vi "GSP_Manager_GT_driver.vi"(4 "error in (no error)":errorcluster, 5 "Grating # (Move Only)":i32, 6 "Action":T1) -> (0 "error out":errorcluster, 3 "reference out (launch only)":refnum<vi>)   [LabVIEW 2015]
doc: "Provides an interface to the Grating Translation Manager. See the actions below.\n\nLaunch - launch the manager thread supplying references to the controls that the thread will update.\n\nHome - Home the grating translation stage\n\nMove - Move the grating to the position supplied by Grating#\n\nShutdown - Shutdown the grating translation manager"
uses:
  GTdriveractions.ctl
  SystemUtil/Command.ctl
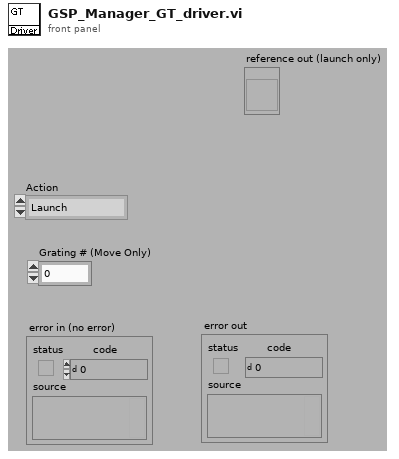
[diagram p1: front panel]
types:
  T1 = typedef "GTdriveractions.ctl" = enum16{"Launch", "INIT_CTL", "Move", "Home", "Shutdown"}
  T2 = typedef "Command.ctl" = cluster{"Command":string, "Parameter":string}
  T3 = cluster{string, "type string":i16[], "data string":string}
  T4 = cluster{string, "type string":i16[], "data string":string}[]
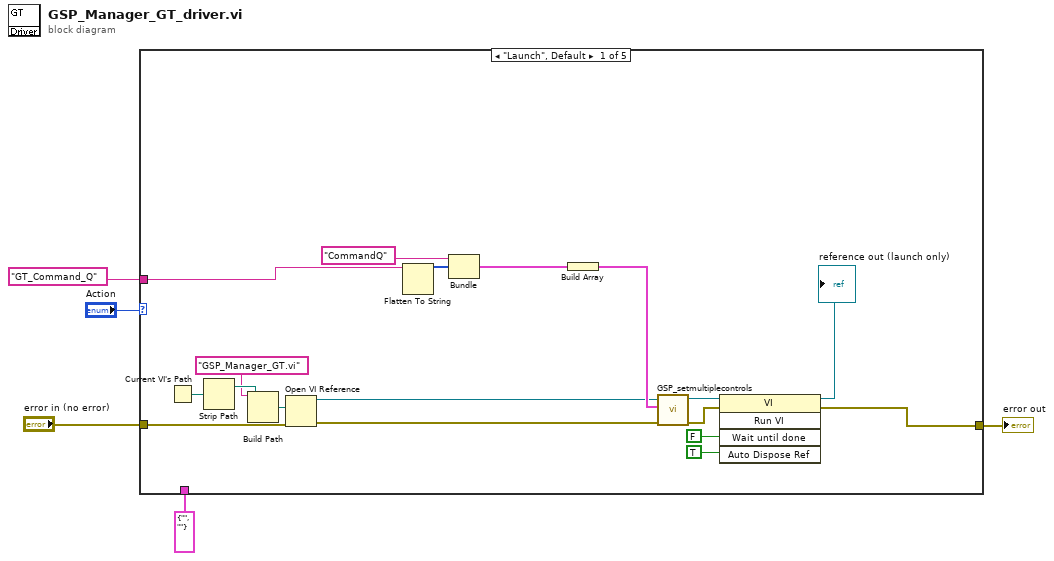
[diagram p0: block diagram]
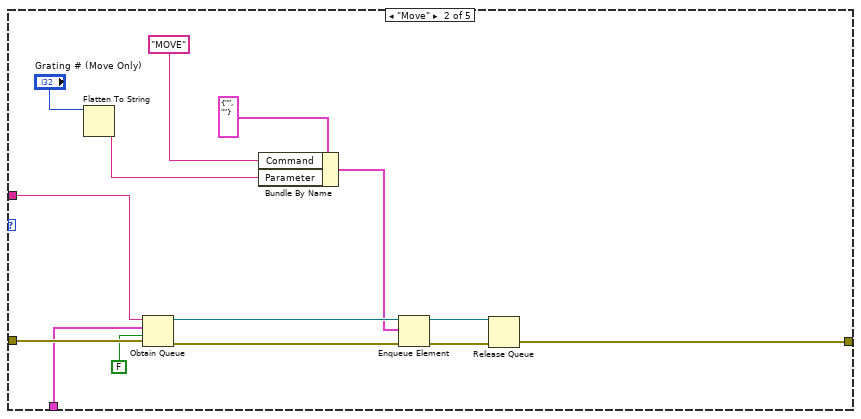
[diagram p2: hidden frame]
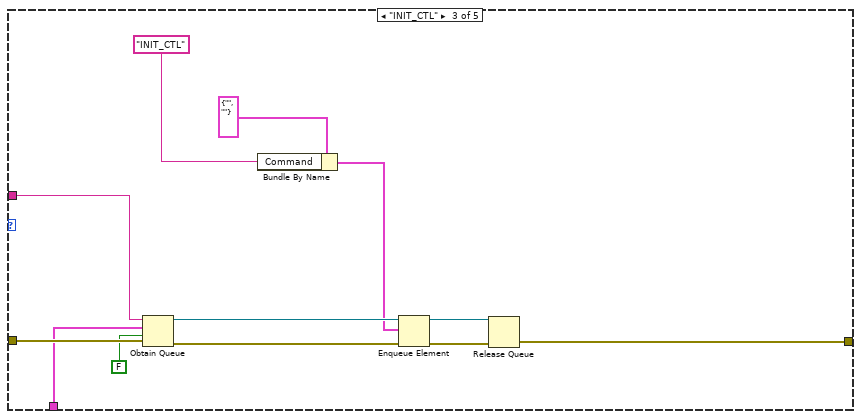
[diagram p3: hidden frame]
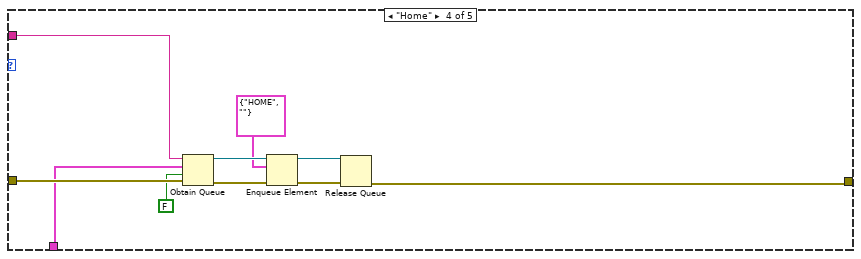
[diagram p4: hidden frame]
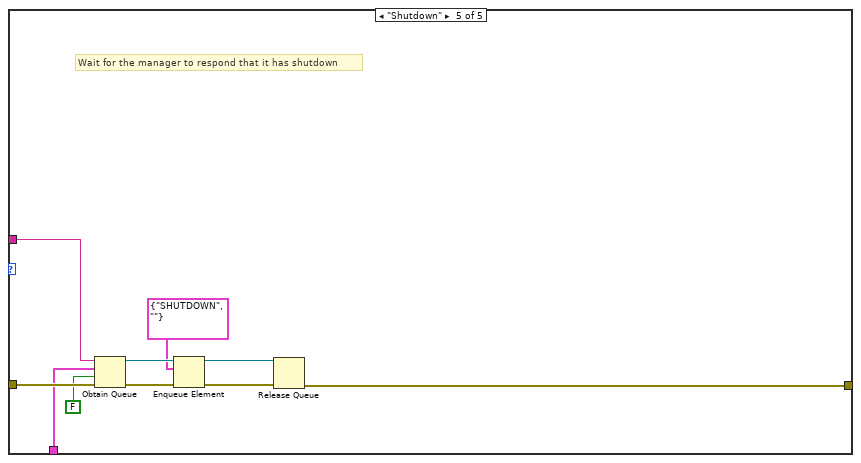
[diagram p5: hidden frame]
diagram:
  n1 = case shown="\"Launch\", Default" "Action" {
    tunnel: "error in (no error)" -> [w20 w38 w50 w58 w70]
    tunnel: [w9 w25 w39 w51 w61] -> w3
    tunnel: "GT_Command_Q" -> [w10 w36 w48 w57 w67]
    tunnel: T2 {"Command"="", "Parameter"=""} ("Command") -> [_ w33 w45 w55 w65]
    frame "Launch", Default {
      n2 = Current VI's Path() -> (path=w14:path)
      n3 = Strip Path(path=w14) -> (stripped path=w12:path)  [unwired: 1 out]
      n4 = Build Path(base path=w12, name or relative path="GSP_Manager_GT.vi" ("vi path")) -> (appended path=w13:path)
      n5 = Open VI Reference(vi path=w13, error in (no error)=w20) -> (vi reference=w8:refnum<vi>, error out=w19:errorcluster)  [unwired: 4 in]
      n6 = Flatten To String(anything=w10) -> (data string=w22:string, type string=w23:i16[])  [unwired: 3 in, 1 out]
      n7 = Bundle("CommandQ", "type string"=w23, "data string"=w22) -> (w7:T3)  [unwired: 1 in]
      n8 = Build Array(w7) -> (w21:T4)
      n9 = call "GSP_setmultiplecontrols.vi"("error in (no error)"=w19, "Control Infos"=w21, "reference"=w8) -> ("error out"=w17:errorcluster, "reference out"=w18:refnum<vi>)  [unwired: 3 in]
      n10 = invoke class="VI" method="Run VI"(reference=w18, error in=w17, "Wait until done"=FALSE, "Auto Dispose Ref"=TRUE) -> (reference out=→"reference out (launch only)":refnum<vi>, error out=w9:errorcluster)  [unwired: 1 in, 3 out]
    }
    frame "Move" {
      n11 = Flatten To String(anything="Grating # (Move Only)") -> (data string=w28:string)  [unwired: 3 in, 2 out]
      n12 = Obtain Queue(name (unnamed)=w36, element data type=w33, create if not found? (T)=FALSE, error in (no error)=w38) -> (queue out=w35:refnum<queue>, error out=w37:errorcluster)  [unwired: 1 in, 1 out]
      n13 = Bundle By Name(cluster=T2 {"Command"="", "Parameter"=""} ("Command"), "Command"="MOVE" ("element"), "Parameter"=w28) -> (w30:T2)
      n14 = Enqueue Element(queue=w35, element=w30, error in (no error)=w37) -> (queue out=w27:refnum<queue>, error out=w26:errorcluster)  [unwired: 1 in, 1 out]
      n15 = Release Queue(queue=w27, error in (no error)=w26) -> (error out=w25:errorcluster)  [unwired: 1 in, 2 out]
    }
    frame "INIT_CTL" {
      n16 = Obtain Queue(name (unnamed)=w48, element data type=w45, create if not found? (T)=FALSE, error in (no error)=w50) -> (queue out=w47:refnum<queue>, error out=w49:errorcluster)  [unwired: 1 in, 1 out]
      n17 = Bundle By Name(cluster=T2 {"Command"="", "Parameter"=""} ("Command"), "Command"="INIT_CTL" ("element")) -> (w42:T2)
      n18 = Enqueue Element(queue=w47, element=w42, error in (no error)=w49) -> (queue out=w41:refnum<queue>, error out=w40:errorcluster)  [unwired: 1 in, 1 out]
      n19 = Release Queue(queue=w41, error in (no error)=w40) -> (error out=w39:errorcluster)  [unwired: 1 in, 2 out]
    }
    frame "Home" {
      n20 = Obtain Queue(name (unnamed)=w57, element data type=w55, create if not found? (T)=FALSE, error in (no error)=w58) -> (queue out=w59:refnum<queue>, error out=w60:errorcluster)  [unwired: 1 in, 1 out]
      n21 = Enqueue Element(queue=w59, element=T2 {"Command"="HOME", "Parameter"=""}, error in (no error)=w60) -> (queue out=w53:refnum<queue>, error out=w52:errorcluster)  [unwired: 1 in, 1 out]
      n22 = Release Queue(queue=w53, error in (no error)=w52) -> (error out=w51:errorcluster)  [unwired: 1 in, 2 out]
    }
    frame "Shutdown" {
      # "Wait for the manager to respond that it has shutdown"
      n23 = Obtain Queue(name (unnamed)=w67, element data type=w65, create if not found? (T)=FALSE, error in (no error)=w70) -> (queue out=w68:refnum<queue>, error out=w69:errorcluster)  [unwired: 1 in, 1 out]
      n24 = Enqueue Element(queue=w68, element=T2 {"Command"="SHUTDOWN", "Parameter"=""}, error in (no error)=w69) -> (queue out=w63:refnum<queue>, error out=w62:errorcluster)  [unwired: 1 in, 1 out]
      n25 = Release Queue(queue=w63, error in (no error)=w62) -> (error out=w61:errorcluster)  [unwired: 1 in, 2 out]
    }
  }
  "error out" <- w3
